vi "Log Critical Error.vi"(8 "error in (no error)":errorcluster, 9 "Critical Error":errorcluster, 10 "Critical Error Event":string, 11 "Trace Controller in":refnum<class "Trace Controller.lvclass">) -> (0 "error out":errorcluster, 3 "Trace Controller out":refnum<class "Trace Controller.lvclass">)   [LabVIEW 2014, in "Robot Actor Framework.lvlib" / "Trace.lvlib" / "Trace Controller.lvclass"]
uses:
  Trace Controller.lvclass
  Trace Controller.lvclass/Trace Controller.ctl
  Utilities/Utilities.lvlib
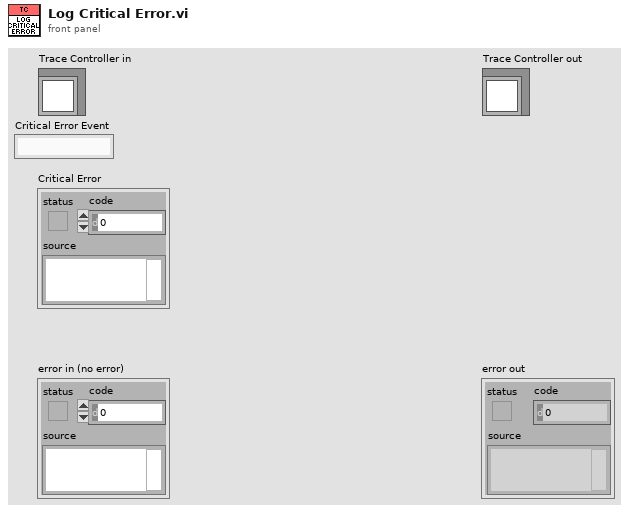
[diagram p1: front panel]
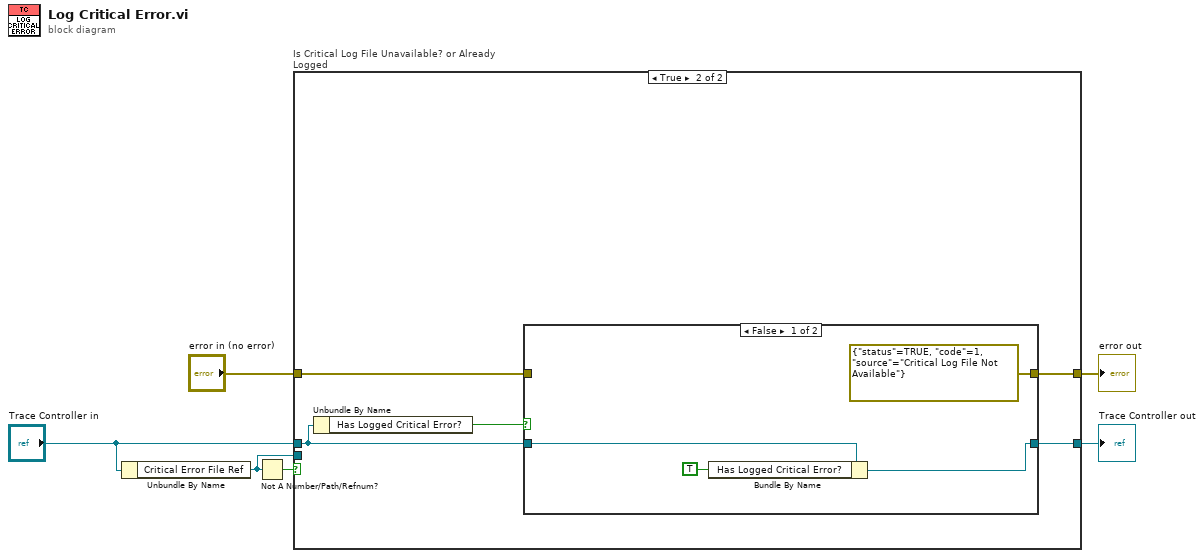
[diagram p0: block diagram]
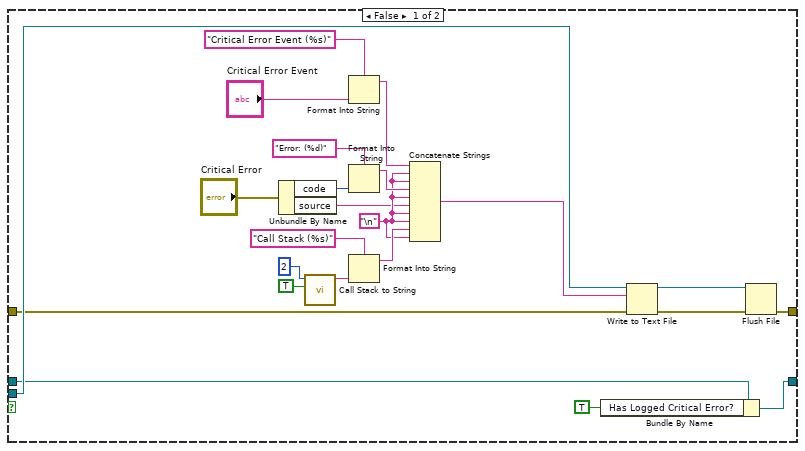
[diagram p2: hidden frame]
diagram:
  n1 = Unbundle By Name("Trace Controller in") -> ("Critical Error File Ref"=w6:refnum<file>)
  n2 = Not A Number/Path/Refnum?(number/path/refnum=w6) -> (NaN/Path/Refnum?=w1:bool)
  n3 = case "Is Critical Log File Unavailable? or Already Logged" shown="True" w1 {
    tunnel: w6 -> [w29 _]
    tunnel: "error in (no error)" -> [w27 w32]
    tunnel: [w25 w34] -> w4
    tunnel: "Trace Controller in" -> [w21 w31]
    tunnel: [w20 w30] -> w2
    frame False {
      w10 = "\n"
      n4 = Unbundle By Name("Critical Error") -> ("code"=w12:i32, "source"=w7:string)
      n5 = call "Call Stack to String.vi"("With EOL Separator"=TRUE, "Call Stacks to Skip"=2) -> ("Call Stack String"=w15:string)  [unwired: 9 in]
      n6 = Format Into String(format string="Critical Error Event (%s)", "Critical Error Event") -> (resulting string=w18:string)  [unwired: 2 in, 1 out]
      n7 = Format Into String(format string="Error: (%d)", w12) -> (resulting string=w11:string)  [unwired: 2 in, 1 out]
      n8 = Format Into String(format string="Call Stack (%s)", w15) -> (resulting string=w14:string)  [unwired: 2 in, 1 out]
      n9 = Concatenate Strings(w18, w10, w10, w11, w10, w7, w10, w10, w14, w10) -> (w17:string)
      n10 = Bundle By Name(cluster=w21, "Has Logged Critical Error?"=TRUE) -> (w20:refnum<class "Trace Controller.lvclass">)
      n11 = Write to Text File(file (use dialog)=w29, text=w17, error in=w27) -> (refnum out=w28:refnum<file>, error out=w26:errorcluster)  [unwired: 1 in, 1 out]
      n12 = Flush File(refnum=w28, error in=w26) -> (error out=w25:errorcluster)  [unwired: 1 out]
    }
    frame True {
      n13 = Unbundle By Name(w31) -> ("Has Logged Critical Error?"=w33:bool)
      n14 = case shown="False" w33 {
        tunnel: [errorcluster {"status"=TRUE, "code"=1, "source"="Critical Log File Not Available"} ("error out") w40] -> w34
        tunnel: w32 -> [_ w40]
        tunnel: w31 -> [w37 w39]
        tunnel: [w36 w39] -> w30
        frame False {
          n15 = Bundle By Name(cluster=w37, "Has Logged Critical Error?"=TRUE) -> (w36:refnum<class "Trace Controller.lvclass">)
        }
        frame True {
        }
      }
    }
  }
  "error out" <- w4
  "Trace Controller out" <- w2
